vi "Neph Server.vi"() -> ()   [LabVIEW 2014]
uses:
  Neph File Observer/Neph File Obs.lvclass
  Nephelometer.lvclass
  Reusable/Session Log/System Log.lvclass
  Reusable/Session APIs/Text Communication/Text Device Session.lvclass
  Reusable/Session APIs/File Access/Config Data/Config Data.lvclass
  Reusable/Session APIs/File Access/Config Data/Config Session.ctl
  Reusable/Session Log/System Log.lvclass/System Log.ctl
  Reusable/Session APIs/File Access/Config Data/Config Data.lvclass/Config Data.ctl
  Reusable/File IO/Class/File Observer.lvclass/File Observer.ctl
  Configurable Device/Configurable Device.lvclass/Configurable Device.ctl
  Nephelometer.lvclass/Nephelometer.ctl
  Reusable/Session APIs/Text Communication/Text Device Session.lvclass/Text Device Session.ctl
  Reusable/Session APIs/Serial/Serial Session.lvclass
  Reusable/Session APIs/File Access/Config Data/Accessors/Write Cfg Path.vi
  Reusable/Session Log/Accessors/Write Main Path.vi
  Reusable/File IO/Class/Accessors/Write Top Data Path.vi
  Reusable/File IO/Class/Accessors/Write File Prefix.vi
  Reusable/File IO/Class/Accessors/Write File Ext.vi
  Reusable/File IO/Class/Accessors/Write File Header.vi
  Reusable/File IO/Class/Accessors/Write Max Size.vi
  Reusable/File IO/Class/Write SwitchonDate_.vi
  Reusable/File IO/Class/Write SwitchonSize_.vi
  Reusable/Session APIs/File Access/Config Data/Accessors/Read Ref.vi
  Configurable Device/Write Handle.vi
  Reusable/Session APIs/Text Communication/Write hSysLog.vi
  Accessors/Write Session Handle.vi
  Read Commands/Get Autozero Mode.vi
  Read Commands/Get Autozero Period.vi
  Read Commands/Get Autozero time.vi
  Unpolled Commands/Set Autozero Period.vi
  Unpolled Commands/Set Autozero Time.vi
  <userlib>/_Session Fwk/Session - Root.lvclass
panel:
  out "Data Record":T1
  out "Auxilary data":T2
  out "Last Zero":timestamp format="%<%H:%M:%S%2u>T"
  in  "New File":bool
  in  "Write":bool
  in  "Zero":bool
  in  "Power":bool
  in  "Heater Power":bool
  in  "ZeroPeriod":u16
  in  "ZeroTime":u16
  in  "AutozeroMode":u8
  out "tremain":i32
  in  "Blower":u8(slide) scale=0.0..255.0
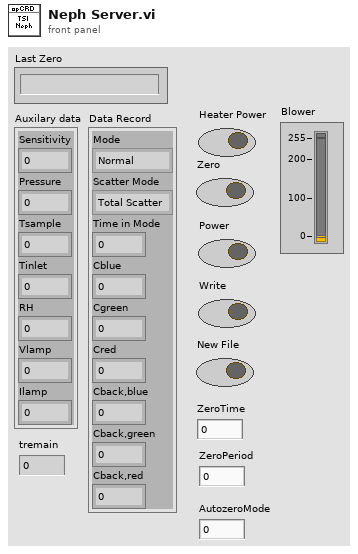
[diagram p1: front panel]
types:
  T1 = cluster{"Mode":enum16{"Normal", "Zero", "Blank"}, "Scatter Mode":enum16{"Total Scatter", "Back Scatter"}, "Time in Mode":i32, "Cblue":dbl, "Cgreen":dbl, "Cred":dbl, "Cback,blue":dbl, "Cback,green":dbl, "Cback,red":dbl}
  T2 = cluster{"Sensitivity":dbl, "Pressure":dbl, "Tsample":dbl, "Tinlet":dbl, "RH":dbl, "Vlamp":dbl, "Ilamp":dbl}
  T3 = typedef "Config Data.lvclass/Config Session.ctl" = refnum<data-value>
  T4 = typedef "Session - Root.lvclass/Session Handle.ctl" = refnum<data-value>
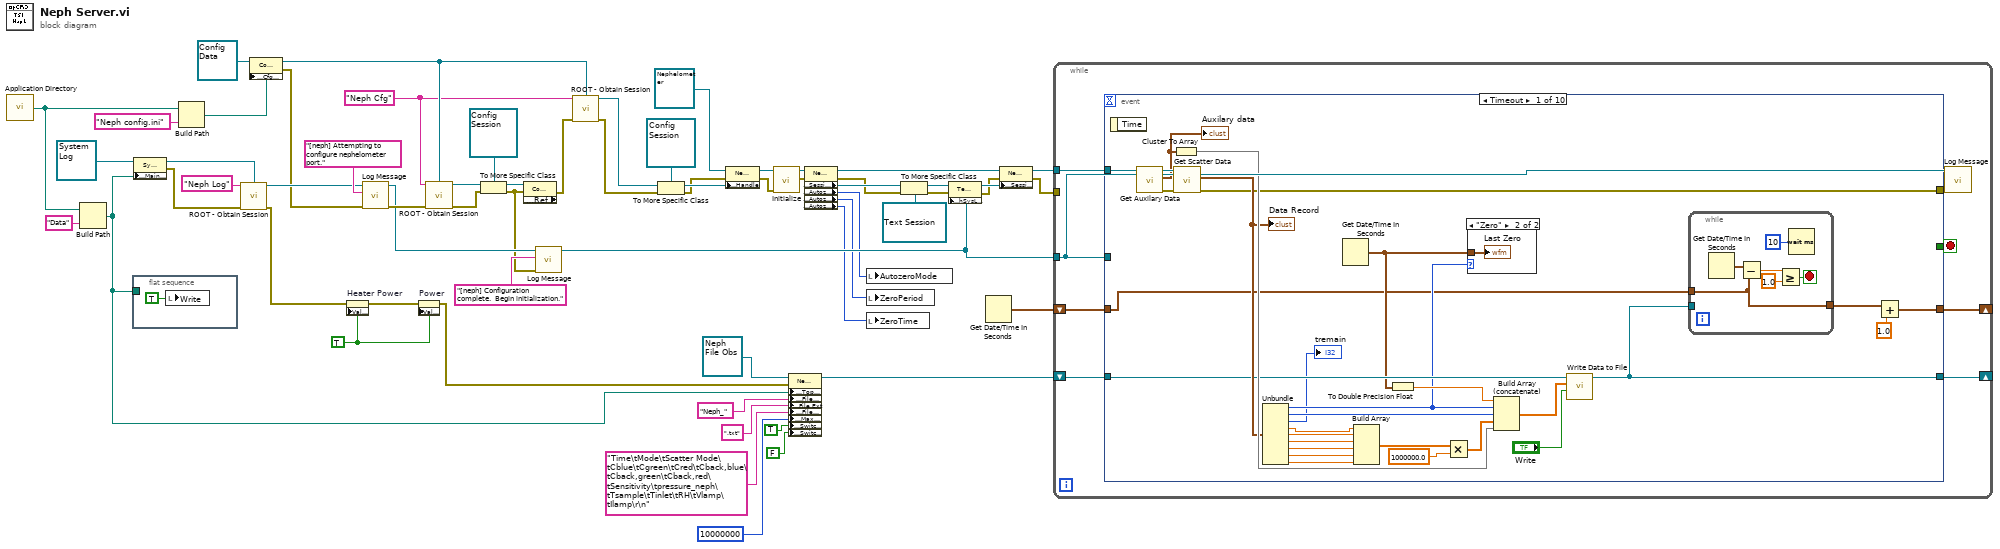
[diagram p0: block diagram]
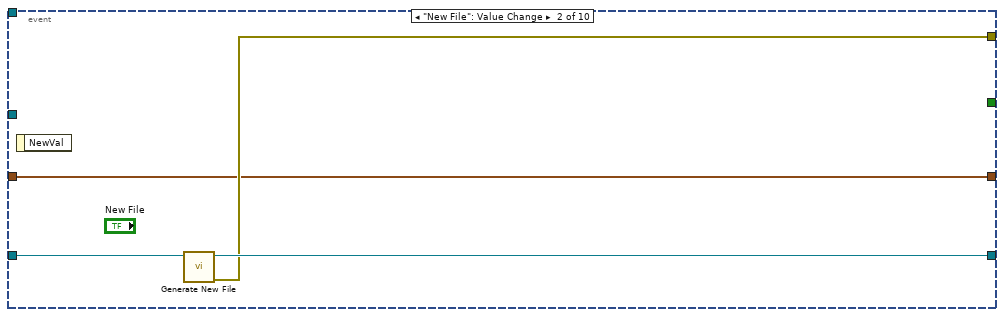
[diagram p3: hidden frame]
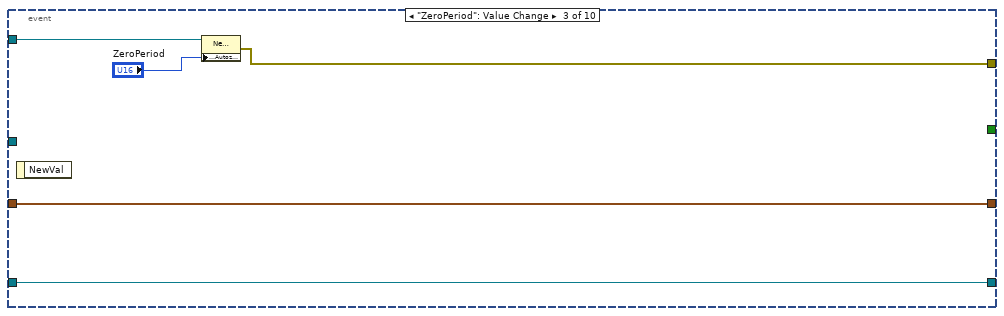
[diagram p4: hidden frame]
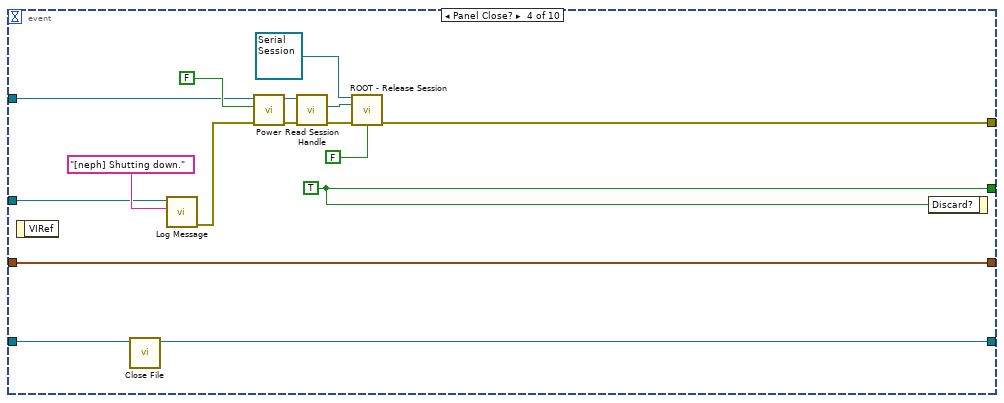
[diagram p5: hidden frame]
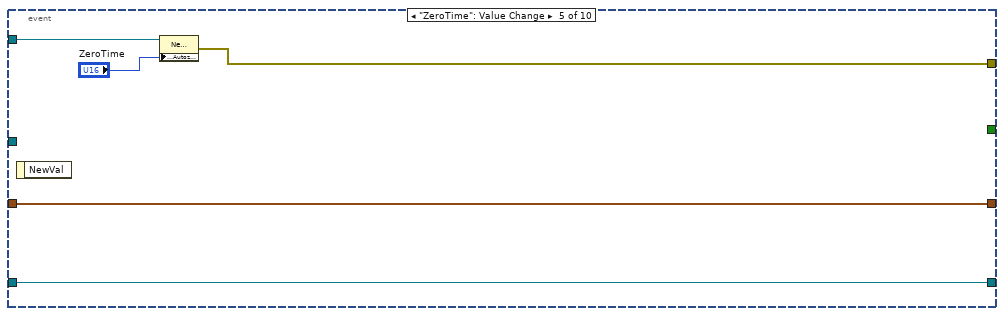
[diagram p6: hidden frame]
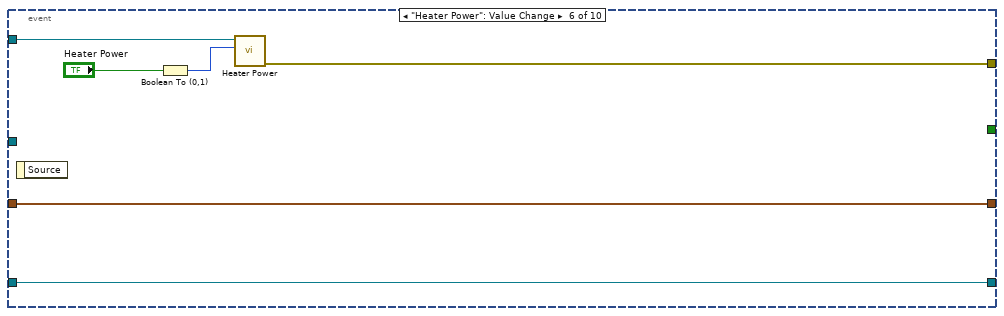
[diagram p7: hidden frame]
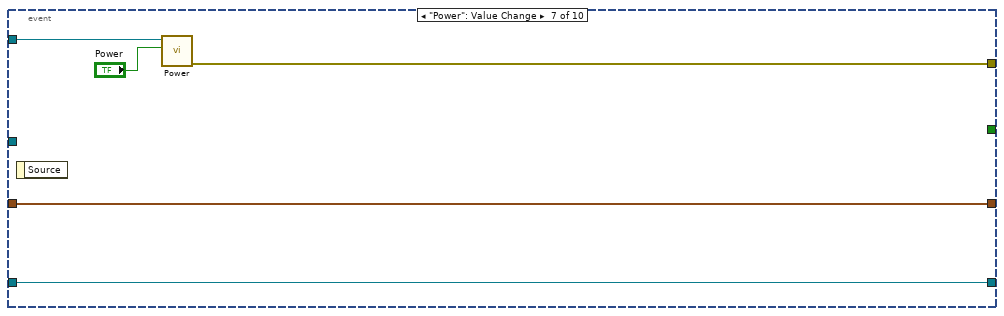
[diagram p8: hidden frame]
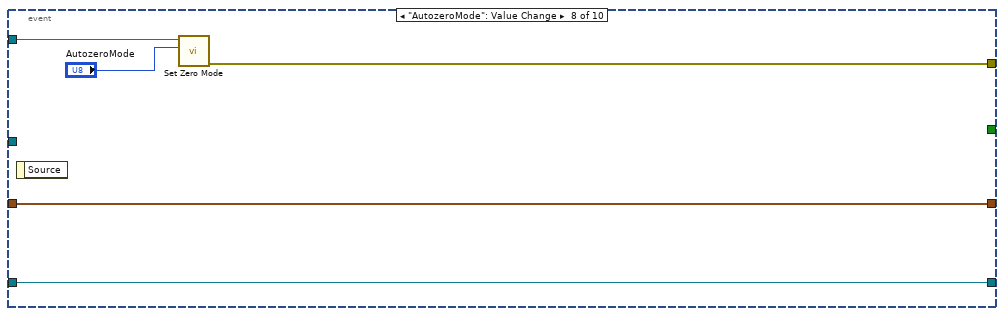
[diagram p9: hidden frame]
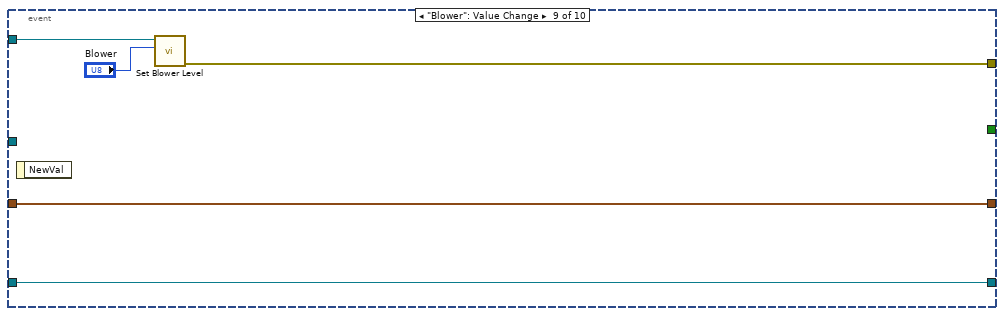
[diagram p10: hidden frame]
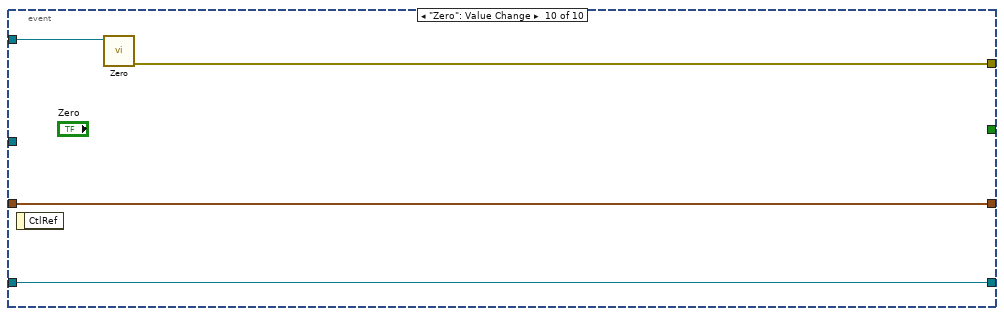
[diagram p11: hidden frame]
diagram:
  w22 = TRUE
  w14 = "Neph Cfg" ("Session Name ()")
  n1 = call <vilib>:"Application Directory.vi"() -> ("Application Directory"=w3:path)
  n2 = Build Path(base path=w3, name or relative path="Data") -> (appended path=w1:path)
  n3 = flat-sequence {
    tunnel: w1 -> [_]
    frame #0 {
      n4 = local write "Write"(TRUE ("Write")) -> ()
    }
  }
  n5 = property class="Sys Log"(reference=refnum<class "System Log.lvclass"> refnum ("Sys Log"), "Accessors:Main Path"=w1) -> (reference out=w41:refnum<class "System Log.lvclass">, error out=w40:errorcluster)  [unwired: 1 in]
  n6 = Build Path(base path=w3, name or relative path="Neph config.ini") -> (appended path=w4:path)
  n7 = call <userlib>:"ROOT - Obtain Session.vi"("Session Name ()"="Neph Log", "OBJ - Session"=w41, "error in (no error)"=w40) -> ("Session Handle"=w38:T4, "error out"=w23:errorcluster)  [unwired: 10 in, 1 out]
  n8 = property class="Config Data"(reference=refnum<class "Config Data.lvclass"> refnum ("Config Data"), "Accessors:Cfg Path"=w4) -> (reference out=w15:refnum<class "Config Data.lvclass">, error out=w16:errorcluster)  [unwired: 1 in]
  n9 = property on="Heater Power" class="Bool (strict)"(error in=w23, "Val(Sgnl)"=w22) -> (error out=w25:errorcluster)  [unwired: 1 in, 1 out]
  n10 = call "Log Message.vi"("error in"=w16, "MSG In"="[neph] Attempting to configure nephelometer port.", "session in"=w38) -> ("error out"=w49:errorcluster, "session out"=w48:T4)  [unwired: 7 in]
  n11 = property on="Power" class="Bool (strict)"(error in=w25, "Val(Sgnl)"=w22) -> (error out=w24:errorcluster)  [unwired: 1 in, 1 out]
  n12 = call <userlib>:"ROOT - Obtain Session.vi"("Session Name ()"=w14, "OBJ - Session"=w15, "error in (no error)"=w49) -> ("Session Handle"=w52:T4, "error out"=w53:errorcluster)  [unwired: 10 in, 1 out]
  n13 = To More Specific Class(target class=T3 refnum ("Session Handle"), reference=w52, error in=w53) -> (specific class reference=w37:T3, error out=w36:errorcluster)
  n14 = property class="Config Data" props=["Accessors:Ref"](reference=w37, error in=w36) -> (error out=w8:errorcluster)  [unwired: 2 out]
  n15 = call "Log Message.vi"("error in"=w36, "MSG In"="[neph] Configuration complete.  Begin initialization.", "session in"=w48) -> ("session out"=w27:T4)  [unwired: 7 in, 1 out]
  n16 = call <userlib>:"ROOT - Obtain Session.vi"("Session Name ()"=w14, "OBJ - Session"=w15, "error in (no error)"=w8) -> ("Session Handle"=w12:T4, "error out"=w7:errorcluster)  [unwired: 10 in, 1 out]
  n17 = To More Specific Class(target class=T3 refnum ("Session Handle"), reference=w12, error in=w7) -> (specific class reference=w11:T3, error out=w9:errorcluster)
  n18 = property class="Neph"(reference=refnum<class "Nephelometer.lvclass"> refnum ("Neph"), error in=w9, "Accessors:Handle"=w11) -> (reference out=w54:refnum<class "Nephelometer.lvclass">, error out=w55:errorcluster)
  n19 = call "Initialize.vi"("error in"=w55, "Neph In"=w54) -> ("error out"=w18:errorcluster, "Neph Out"=w56:refnum<class "Nephelometer.lvclass">)  [unwired: 8 in]
  n20 = property class="Neph File Obs"(reference=refnum<class "Neph File Obs.lvclass"> refnum ("Neph File Obs"), error in=w24, "Data Access:Top Data Path"=w1, "Data Access:File Prefix"="Neph_" ("File Prefix"), "Data Access:File Ext"=".txt" ("File Ext"), "Data Access:File Header"="Time\tMode\tScatter Mode\tCblue\tCgreen\tCred\tCback,blue\tCback,green\tCback,red\tSensitivity\tpressure_neph\tTsample\tTinlet\tRH\tVlamp\tIlamp\r\n" ("File Header"), "Data Access:Max Size"=i64 10000000 ("Max Size"), "Accessors:SwitchonDate_"=TRUE ("SwitchonDate_"), "Accessors:SwitchonSize_"=FALSE ("SwitchonSize_")) -> (reference out=w26:refnum<class "Neph File Obs.lvclass">)  [unwired: 1 out]
  n21 = property class="Neph"(reference=w56, error in=w18) -> (reference out=w46:refnum<class "Nephelometer.lvclass">, error out=w32:errorcluster, "Accessors:Session Handle"=w35:T4, "Commands:Autozero Mode"=w21:u8, "Commands:Autozero Period"=w20:u16, "Commands:Autozero Time"=w19:u16)
  n22 = local write "AutozeroMode"(w21) -> ()
  n23 = local write "ZeroPeriod"(w20) -> ()
  n24 = local write "ZeroTime"(w19) -> ()
  n25 = To More Specific Class(target class=refnum<data-value> refnum ("Session Handle"), reference=w35, error in=w32) -> (specific class reference=w33:refnum<data-value>, error out=w31:errorcluster)
  n26 = property class="Text Session"(reference=w33, error in=w31, "Accessors:hSysLog"=w27) -> (reference out=w45:refnum<data-value>, error out=w43:errorcluster)
  n27 = Get Date/Time In Seconds() -> (seconds since 1Jan1904=w6:timestamp)
  n28 = property class="Neph"(reference=w46, error in=w43, "Accessors:Session Handle"=w45) -> (reference out=w28:refnum<class "Nephelometer.lvclass">, error out=w10:errorcluster)
  n29 = while {
    tunnel: w28 -> [w70]
    tunnel: w27 -> [w65]
    shift-right: [w67] -> _
    shift-left: w26 -> [w68]
    tunnel: w10 -> [_]
    shift-right: [w63] -> _
    shift-left: w6 -> [w64]
    stop <- w69 stop-if-true
    n30 = event shown="[0] Timeout" {
      selector: _ -> [_ _ _ _ _ _ _ _ _ _]
      dyn-events: _ -> [_ _ _ _ _ _ _ _ _ _]
      timeout: _ -> [_ _ _ _ _ _ _ _ _ _]
      tunnel: w70 -> [w99 _ w115 w122 w135 w140 w146 w151 w157 w161]
      tunnel: [_ _ _ w131 _ _ _ _ _ _] -> w69
      tunnel: w68 -> [w84 w110 w113 w130 w136 w139 w145 w149 w155 w160]
      tunnel: [w75 w109 w113 w129 w136 w139 w145 w149 w155 w160] -> w67
      tunnel: [w81 w108 w112 w120 w133 w138 w144 w150 w154 w159] -> w66
      tunnel: w65 -> [_ _ _ w118 _ _ _ _ _ _]
      tunnel: w64 -> [w74 w107 w111 w116 w132 w137 w143 w148 w153 w158]
      tunnel: [w71 w107 w111 w116 w132 w137 w143 w148 w153 w158] -> w63
      event Timeout {
        n31 = event-data() -> ()  [unwired: 1 in, 1 out]
        n32 = call "Get Auxilary Data.vi"("Neph in"=w99) -> ("error out"=w80:errorcluster, "Auxilary data"=w89:T2, "Neph out"=w98:refnum<class "Nephelometer.lvclass">)  [unwired: 8 in]
        "Auxilary data" <- w89
        n33 = Cluster To Array(cluster=w89) -> (array=w90:dbl[])
        n34 = call "Get Scatter Data.vi"("error in"=w80, "Neph in"=w98) -> ("error out"=w81:errorcluster, "Data Record"=w88:T1)  [unwired: 7 in, 1 out]
        "Data Record" <- w88
        n35 = Unbundle(w88) -> ("Mode"=w79:enum16{"Normal", "Zero", "Blank"}, "Scatter Mode"=w97:enum16{"Total Scatter", "Back Scatter"}, "Time in Mode"=→"tremain":i32, "Cblue"=w96:dbl, "Cgreen"=w95:dbl, "Cred"=w94:dbl, "Cback,blue"=w93:dbl, "Cback,green"=w87:dbl, "Cback,red"=w86:dbl)
        n36 = Get Date/Time In Seconds() -> (seconds since 1Jan1904=w78:timestamp)
        n37 = Build Array(w96, w95, w94, w93, w87, w86) -> (w92:dbl[])
        n38 = To Double Precision Float(number=w78) -> (double precision float=w82:dbl)
        n39 = Multiply(x=w92, y=1000000.0 ("Cback,red")) -> (x*y=w91:dbl[])
        n40 = case shown="\"Zero\"" w79 {
          tunnel: w78 -> [_ w106]
          frame "Normal", Default {
          }
          frame "Zero" {
            "Last Zero" <- w106
          }
        }
        n41 = Build Array (concatenate)(w82, w79, w97, w91, w90) -> (w83:dbl[])
        n42 = call "Write Data to File.vi"("Write?"="Write", "Data In"=w83, "Neph File Obs in"=w84) -> ("Neph File Obs out"=w75:refnum<class "Neph File Obs.lvclass">)  [unwired: 7 in, 1 out]
        n43 = while {
          tunnel: w75 -> [_]
          tunnel: w74 -> [w101]
          tunnel: [w101] -> w73
          stop <- w102 stop-if-true
          n44 = Get Date/Time In Seconds() -> (seconds since 1Jan1904=w105:timestamp)
          n45 = Subtract(x=w105, y=w101) -> (x-y=w104:dbl)
          n46 = Greater Or Equal?(x=w104, y=1.0) -> (x >= y?=w102:bool)
          n47 = Wait (ms)(milliseconds to wait=u32 10) -> ()  [unwired: 1 out]
        }
        n48 = Add(x=w73, y=1.0) -> (x+y=w71:timestamp)
      }
      event "New File": Value Change {
        n49 = event-data() -> ()  [unwired: 1 in, 1 out]
        n50 = call-dynamic "Generate New File.vi"("File Obs in"=w110) -> ("error out"=w108:errorcluster, "File Obs out"=w109:refnum<class "Neph File Obs.lvclass">)  [unwired: 8 in, 1 out]
      }
      event "ZeroPeriod": Value Change {
        n51 = event-data() -> ()  [unwired: 1 in, 1 out]
        n52 = property class="Neph"(reference=w115, "Commands:Autozero Period"="ZeroPeriod") -> (error out=w112:errorcluster)  [unwired: 1 in, 1 out]
      }
      event Panel Close? {
        w131 = TRUE ("Discard?")
        n53 = event-data() -> ()  [unwired: 1 in, 1 out]
        n54 = call-dynamic "Close File.vi"("File Obs in"=w130) -> ("File Obs out"=w129:refnum<class "Neph File Obs.lvclass">)  [unwired: 9 in, 1 out]
        n55 = call "Log Message.vi"("MSG In"="[neph] Shutting down.", "session in"=w118) -> ("error out"=w117:errorcluster)  [unwired: 8 in, 1 out]
        n56 = call "Power.vi"("error in"=w117, "Power?"=FALSE, "Neph in"=w122) -> ("error out"=w125:errorcluster, "Neph out"=w124:refnum<class "Nephelometer.lvclass">)  [unwired: 7 in]
        n57 = call "Read Session Handle.vi"("error in (no error)"=w125, "Nephelometer in"=w124) -> ("error out"=w121:errorcluster, "Session Handle"=w127:T4)  [unwired: 7 in, 1 out]
        n58 = call <userlib>:"ROOT - Release Session.vi"("OBJ - Session in"=refnum<class "Serial Session.lvclass"> refnum ("Serial Session"), "Session Handle in"=w127, "error in (no error)"=w121, "force destroy? (F)"=FALSE) -> ("error out"=w120:errorcluster)  [unwired: 10 in, 1 out]
        n59 = event-data("Discard?"=w131) -> ()  [unwired: 1 in, 1 out]
      }
      event "ZeroTime": Value Change {
        n60 = event-data() -> ()  [unwired: 1 in, 1 out]
        n61 = property class="Neph"(reference=w135, "Commands:Autozero Time"="ZeroTime") -> (error out=w133:errorcluster)  [unwired: 1 in, 1 out]
      }
      event "Heater Power": Value Change {
        n62 = event-data() -> ()  [unwired: 1 in, 1 out]
        n63 = Boolean To (0,1)(Boolean="Heater Power") -> (0, 1=w142:i16)
        n64 = call "Heater Power.vi"("On/Off"=w142, "Neph in"=w140) -> ("error out"=w138:errorcluster)  [unwired: 8 in, 1 out]
      }
      event "Power": Value Change {
        n65 = event-data() -> ()  [unwired: 1 in, 1 out]
        n66 = call "Power.vi"("Power?"="Power", "Neph in"=w146) -> ("error out"=w144:errorcluster)  [unwired: 8 in, 1 out]
      }
      event "AutozeroMode": Value Change {
        n67 = event-data() -> ()  [unwired: 1 in, 1 out]
        n68 = call "Set Zero Mode.vi"("Mode"="AutozeroMode", "Neph in"=w151) -> ("error out"=w150:errorcluster)  [unwired: 8 in, 1 out]
      }
      event "Blower": Value Change {
        n69 = event-data() -> ()  [unwired: 1 in, 1 out]
        n70 = call "Set Blower Level.vi"("Level"="Blower", "Neph in"=w157) -> ("error out"=w154:errorcluster)  [unwired: 8 in, 1 out]
      }
      event "Zero": Value Change {
        n71 = event-data() -> ()  [unwired: 1 in, 1 out]
        n72 = call "Zero.vi"("Neph in"=w161) -> ("error out"=w159:errorcluster)  [unwired: 9 in, 1 out]
      }
    }
    n73 = call "Log Message.vi"("error in"=w66, "session in"=w65) -> ()  [unwired: 8 in, 2 out]
  }
